vi "Decoder.vi"(11 "Input":string) -> (3 "Data":sgl[](array[numeric]))   [LabVIEW 2010, in "DPR250.lvlib"]
uses:
  DPR250.lvlib
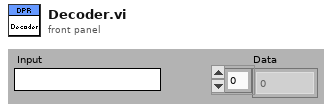
[diagram p1: front panel]
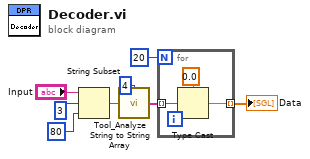
[diagram p0: block diagram]
diagram:
  n1 = String Subset(string="Input", offset (0)=3, length (rest)=80 ("length (rest)")) -> (substring=w4:string)
  n2 = call "Tool_Analyze String to String Array.vi"("Length (1)"=4, "String"=w4) -> ("String Array"=w2:string[])  [unwired: 13 in]
  n3 = for {
    N: 20 -> [_]
    tunnel: w2 -> [w11] mode=indexing
    tunnel: [w9] -> w8 mode=indexing
    n4 = Type Cast(type=sgl 0.0, x=w11) -> (*(type *) &x=w9:sgl)
  }
  "Data" <- w8
